vi "BLIP on True.vi"(1 "Boolean Input":bool) -> (0 "Blip on True":bool)   [LabVIEW 2018]
doc: "This VI crates a \"Blip\", or a fast pulse, upon receiving a False to True transition. In other words, when something goes \"True\" or \"High\", this will supply a fast pulse, which can be used to trigger events that do not want a constant signal. \n\n{{{{ RDS }}}}"
panel:
  # "BLIP on TRUE"
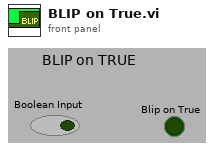
[diagram p1: front panel]
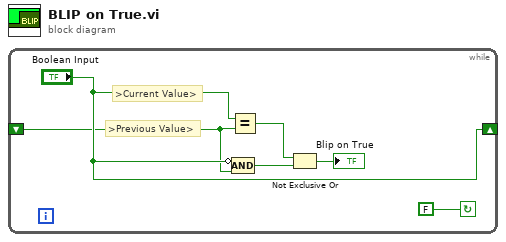
[diagram p0: block diagram]
diagram:
  n1 = while {
    shift-left: _ -> [w3]
    shift-right: ["Boolean Input"] -> _
    stop <- FALSE continue-if-true
    # ">Current Value>"
    # ">Previous Value>"
    n2 = Equal?(x="Boolean Input", y=w3) -> (x = y?=w5:bool)
    n3 = Compound Arithmetic op=AND(invert "Boolean Input", w3) -> (w2:bool)
    n4 = Not Exclusive Or(1:w2, 2:w5) -> (0:→"Blip on True":bool)
  }
